vi "TCP-IP Server.vi"() -> ()   [LabVIEW 2020, in "Startup Processes.lvlib"]
doc: "This VI acts as a server for an incoming websockets connection. Receives/sends string data to the connected client.\nWebSockets API 1.3.0.13\nSam Sharp - Intelligent Energy\nCopyright (c) 2015, Intelligent Energy"
uses:
  Startup Processes.lvlib
  _typedefs/TCPIP Listener States.ctl
  toolbox/Standard Signalling/ude_Stop Application/Get Event Reference.vi
  toolbox/Standard Signalling/ude_Stop Application/ude_Stop Application.lvlib
  toolbox/Standard Signalling/ude_Handle Errors/ude_Handle Errors.lvlib
panel:
  out "Port Number":u32
  out "Connected to...":string
  out "Last Connection":timestamp
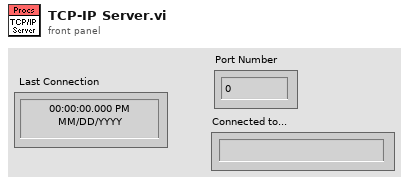
[diagram p1: front panel]
types:
  T1 = typedef "Startup Processes.lvlib/TCPIP Listener States.ctl" = enum16{"Initialize Listener", "Wait For Connection", "Spawn Handler", "Close Listener"}
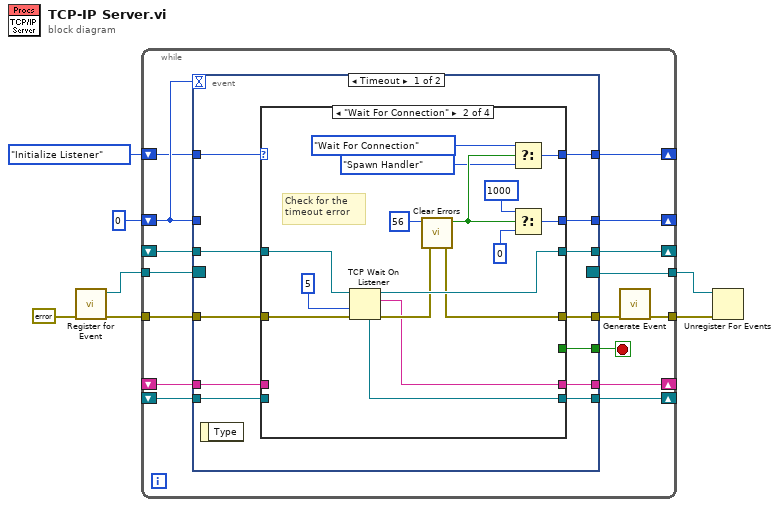
[diagram p0: block diagram]
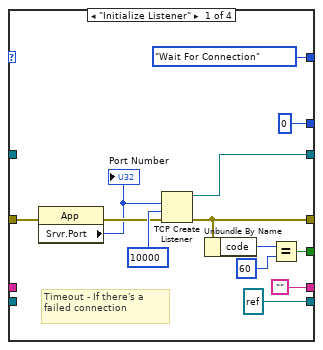
[diagram p2: hidden frame]
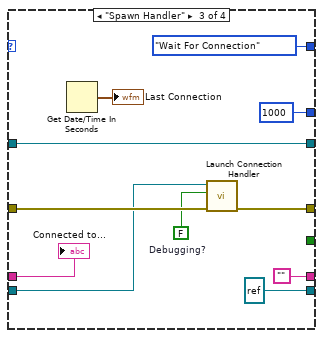
[diagram p3: hidden frame]
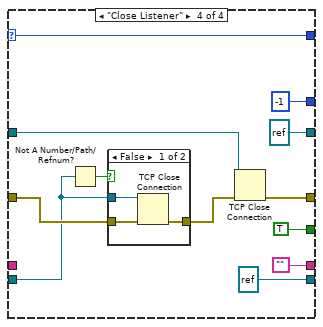
[diagram p4: hidden frame]
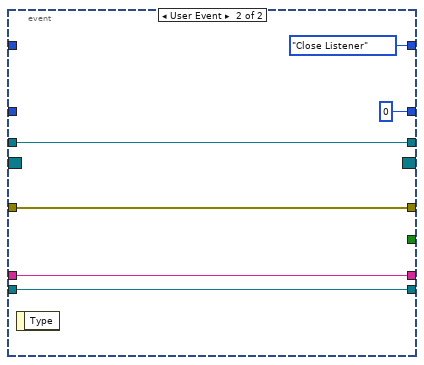
[diagram p6: hidden frame]
diagram:
  n1 = call "Register for Event.vi"("Error In"=errorcluster {"status"=FALSE, "code"=0, "source"=""} ("Error Out")) -> ("Error Out"=w3:errorcluster, "sys"=w2:refnum<event-registration>)  [unwired: 5 in]
  n2 = while {
    shift-right: [w21] -> _
    shift-left: _ -> [w23]
    shift-right: [w18] -> _
    shift-left: 0 -> [w20]
    shift-right: [w17] -> _
    shift-left: _ -> [w16]
    shift-right: [w14] -> _
    shift-left: TCPIP_Listener_States."Initialize Listener" -> [w15]
    tunnel: w3 -> [w22]
    tunnel: [w10] -> w5
    tunnel: w2 -> [w13]
    tunnel: [w12] -> w1
    shift-right: [w9] -> _
    shift-left: _ -> [w8]
    stop <- w19 stop-if-true
    n3 = event shown="[0] Timeout" {
      selector: w13 -> [_ _]
      dyn-events: [_ _] -> w12
      timeout: w20 -> [_ _]
      tunnel: w23 -> [w35 w94]
      tunnel: w22 -> [w34 w93]
      tunnel: [w33 w94] -> w21
      tunnel: [w32 w93] -> w11
      tunnel: w20 -> [_ _]
      tunnel: [w31 _] -> w19
      tunnel: [w30 0] -> w18
      tunnel: [w29 w97] -> w17
      tunnel: w16 -> [w28 w97]
      tunnel: w15 -> [w27 _]
      tunnel: [w26 TCPIP_Listener_States."Close Listener"] -> w14
      tunnel: [w25 w92] -> w9
      tunnel: w8 -> [w24 w92]
      event Timeout {
        n4 = event-data() -> ()  [unwired: 1 in, 1 out]
        n5 = case shown="\"Wait For Connection\"" w27 {
          selector: w27 -> [_ _ _ w87]
          tunnel: w35 -> [_ w64 w74 w84]
          tunnel: w34 -> [w44 w63 w73 w80]
          tunnel: [w45 w62 w74 refnum<k5> refnum ("listener ID")] -> w33
          tunnel: [w39 w58 w72 w83] -> w32
          tunnel: [w38 _ _ TRUE ("status")] -> w31
          tunnel: [0 w57 1000 ("t") -1 ("t")] -> w30
          tunnel: [refnum<k5> refnum ("listener ID") w55 refnum<k5> refnum ("listener ID") refnum<k5> refnum ("listener ID")] -> w29
          tunnel: w28 -> [_ _ w68 w78]
          tunnel: [TCPIP_Listener_States."Wait For Connection" w53 TCPIP_Listener_States."Wait For Connection" w87] -> w26
          tunnel: ["" w49 "" ""] -> w25
          tunnel: w24 -> [_ _ w66 _]
          frame "Initialize Listener" {
            # "Timeout - If there's a failed connection"
            n6 = property class="App"(error in=w44) -> (error out=w43:errorcluster, "Srvr.Port"=w41:u32)  [unwired: 1 in, 1 out]
            "Port Number" <- w41
            n7 = TCP Create Listener(8:w43, 9:10000 ("timeout ms (25000)"), 10:w41) -> (0:w39:errorcluster, 3:w45:refnum<k5>)  [unwired: 2 in, 1 out]
            n8 = Unbundle By Name(w39) -> ("code"=w37:i32)
            n9 = Equal?(x=w37, y=60) -> (x = y?=w38:bool)
          }
          frame "Wait For Connection" {
            # "Check for the timeout error"
            n10 = TCP Wait On Listener(8:w63, 9:5 ("timeout ms (wait forever: -1)"), 11:w64) -> (0:w59:errorcluster, 2:w49:string, 3:w62:refnum<k5>, 4:w55:refnum<k5>)  [unwired: 1 in, 1 out]
            n11 = call <vilib>:"Clear Errors.vi"("error in (no error)"=w59, "specific error code to clear (0: all)"=56) -> ("error out"=w58:errorcluster, "specific error cleared?"=w52:bool)  [unwired: 4 in]
            n12 = Select(t=TCPIP_Listener_States."Wait For Connection", s=w52, f=TCPIP_Listener_States."Spawn Handler") -> (s? t:f=w53:T1)
            n13 = Select(t=1000, s=w52, f=0) -> (s? t:f=w57:i32)
          }
          frame "Spawn Handler" {
            w71 = FALSE  # Debugging?
            n14 = Get Date/Time In Seconds() -> (seconds since 1Jan1904=→"Last Connection":timestamp)
            n15 = call "Launch Connection Handler.vi"("error in (no error)"=w73, "Debugging?"=w71, "TCP Network Connection in"=w68) -> ("error out"=w72:errorcluster)  [unwired: 4 in]
            "Connected to..." <- w66
          }
          frame "Close Listener" {
            n16 = Not A Number/Path/Refnum?(number/path/refnum=w78) -> (NaN/Path/Refnum?=w77:bool)
            n17 = case shown="False" w77 {
              tunnel: w80 -> [w90 w91]
              tunnel: [w89 w91] -> w79
              tunnel: w78 -> [w88 _]
              frame False {
                n18 = TCP Close Connection(connection ID=w88, error in (no error)=w90) -> (error out=w89:errorcluster)  [unwired: 1 in, 1 out]
              }
              frame True {
              }
            }
            n19 = TCP Close Connection(connection ID=w84, error in (no error)=w79) -> (error out=w83:errorcluster)  [unwired: 1 in, 1 out]
          }
        }
      }
      event User Event {
        n20 = event-data() -> ()  [unwired: 1 in, 1 out]
      }
    }
    n21 = call "Generate Event.vi"("Error In"=w11) -> ("Error Out"=w10:errorcluster)  [unwired: 6 in]
  }
  n22 = Unregister For Events(event registration refnum=w1, error in=w5) -> ()  [unwired: 1 out]
